vi "end time 2.0.vi"(2 "start":u32, 3 "unit":u32, 4 "End time":dbl) -> (0 "Boolean":bool, 1 "dt ideale":dbl)   [LabVIEW 2012]
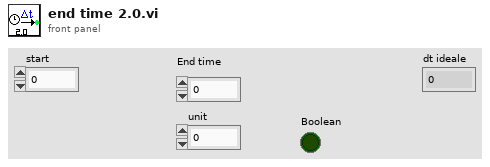
[diagram p1: front panel]
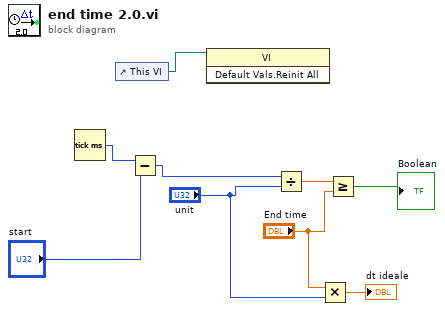
[diagram p0: block diagram]
diagram:
  n1 = Tick Count (ms)() -> (millisecond timer value=w8:u32)
  n2 = control-ref of="This VI"() -> (w4:refnum<vi>)
  n3 = Subtract(x=w8, y="start") -> (x-y=w7:u32)
  n4 = invoke class="VI" method="Default Vals.Reinit All"(reference=w4) -> ()  [unwired: 2 in, 3 out]
  n5 = Divide(x=w7, y="unit") -> (x/y=w9:dbl)
  n6 = Multiply(x="End time", y="unit") -> (x*y=→"dt ideale":dbl)
  n7 = Greater Or Equal?(x=w9, y="End time") -> (x >= y?=→"Boolean":bool)
